vi "get_galvo_voltages.vi"(8 "error in (no error)":errorcluster, 11 "ImagingModeDL090130Frame in":refnum<class "ImagingModeDL090130Frame.lvclass">) -> (0 "error out":errorcluster, 1 "deltaVy(V)":dbl, 2 "Vy0(V)":dbl, 3 "ImagingModeDL090130Frame out":refnum<class "ImagingModeDL090130Frame.lvclass">, 4 "Vz0(V)":dbl, 6 "deltaVz(V)":dbl)   [LabVIEW 2010, in "ImagingModeDL090130Frame.lvclass"]
uses:
  ImagingModeDL090130Frame.lvclass
  ImagingModeDL090130Frame.lvclass/ImagingModeDL090130Frame.ctl
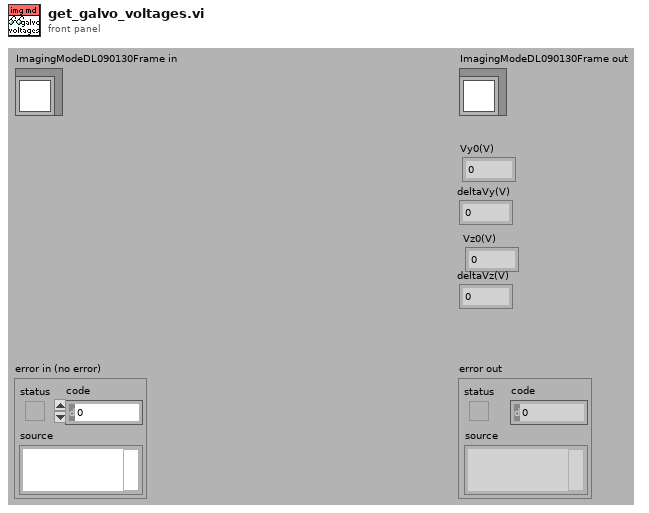
[diagram p1: front panel]
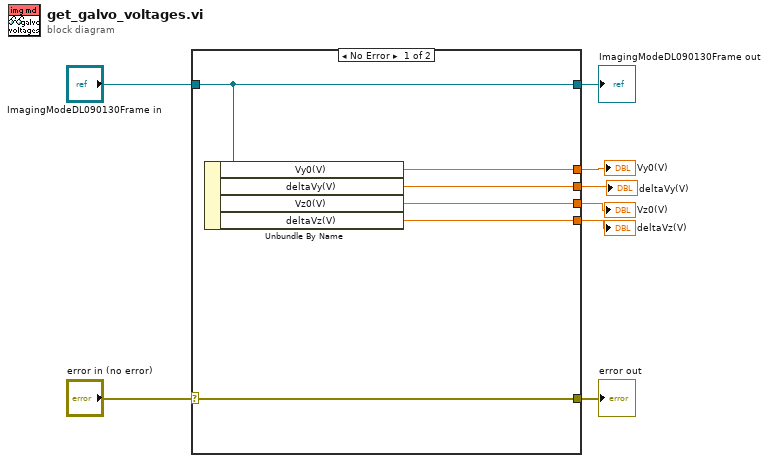
[diagram p0: block diagram]
diagram:
  n1 = case shown="No Error" "error in (no error)" {
    selector: "error in (no error)" -> [w14 w15]
    tunnel: [w14 w15] -> w7
    tunnel: [w13 w16] -> w5
    tunnel: "ImagingModeDL090130Frame in" -> [w13 w16]
    tunnel: [w12 _] -> w4
    tunnel: [w11 _] -> w3
    tunnel: [w10 _] -> w2
    tunnel: [w9 _] -> w1
    frame No Error {
      n2 = Unbundle By Name(w13) -> ("Vy0(V)"=w12:dbl, "deltaVy(V)"=w11:dbl, "Vz0(V)"=w10:dbl, "deltaVz(V)"=w9:dbl)
    }
    frame Error {
    }
  }
  "error out" <- w7
  "ImagingModeDL090130Frame out" <- w5
  "Vy0(V)" <- w4
  "deltaVy(V)" <- w3
  "Vz0(V)" <- w2
  "deltaVz(V)" <- w1
